vi "KN-StringTo矩形AndOptions.vi"(0 "String":string) -> (4 "ROI Descriptor":T5 {"Contours"."Type" items=["No Selection", "Point", "Line", "Rectangle", "Oval", "Polygon", "Freehand Region", "Annulus", "Unused2", "Unused3", "Broken Line", "Freehand Line", "Rotated Rectangle"]}, 6 "Option All":T4 {"Edge Options"."Edge Polarity" items=["All Edges", "Rising Edges", "Falling Edges"]; "Edge Options"."Minimum Edge Strength" format="%.2f"; "Edge Options"."Width" step=2; "Edge Options"."Kernel Size" step=2}, 8 "UI SHOW":T3 {"Edge Options"."Edge Polarity" items=["All Edges", "Rising Edges", "Falling Edges"]; "Edge Options"."Minimum Edge Strength" format="%.2f"; "Edge Options"."Width" step=2; "Edge Options"."Kernel Size" step=2}, 15 "Range (Threshold 1)":cluster{"Lower value":sgl, "Upper value":sgl}={"Lower value"=218.0, "Upper value"=255.0})   [LabVIEW 2015]
uses:
  <vilib>/vision/Measure.llb/Edge Options.ctl
  <vilib>/vision/Measure.llb/Edge Polarity.ctl
panel:
  out "已删除元素的数组子集":string[](array[string])
  out "已删除的部分":string[](array[string])
  out "All Data":string[](array[string])
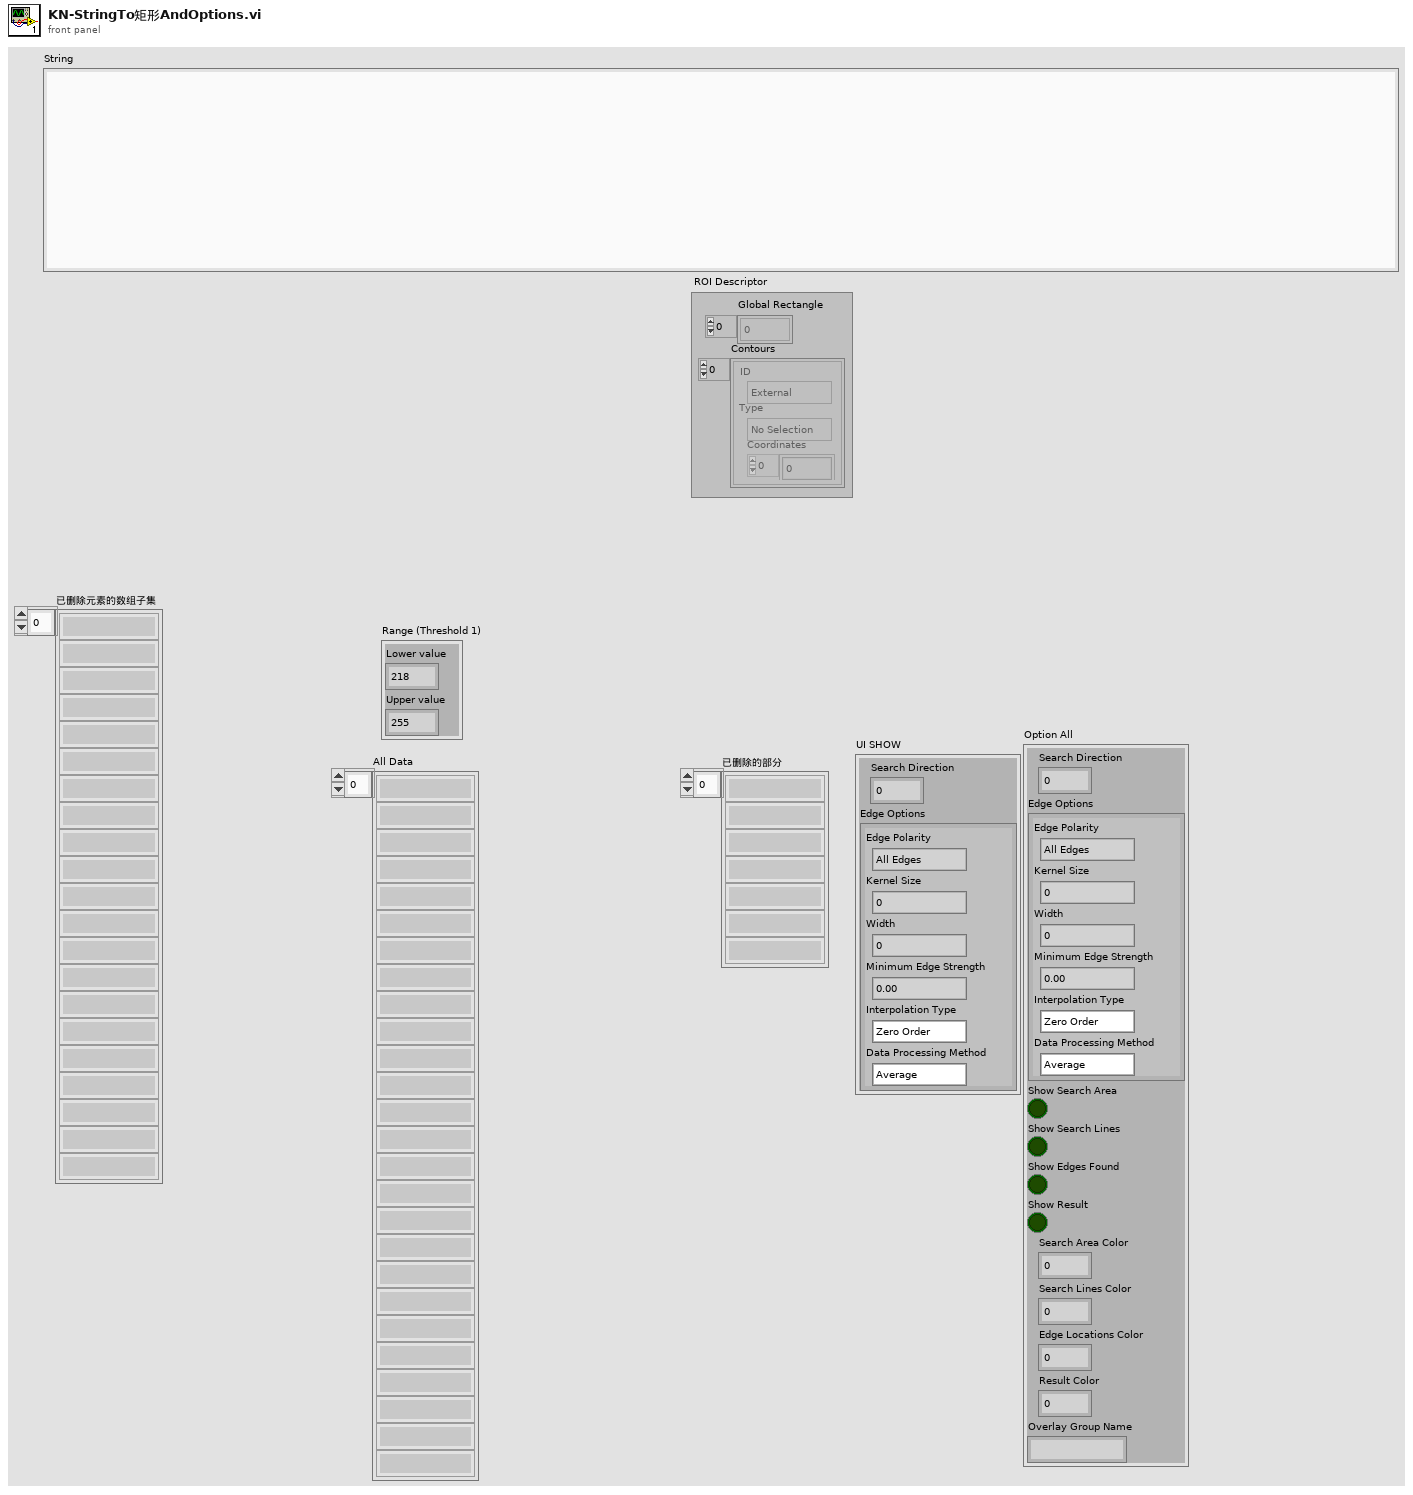
[diagram p1: front panel]
types:
  T1 = typedef "Edge Options.ctl" = cluster{"Edge Polarity":T2, "Kernel Size":u32, "Width":u32, "Minimum Edge Strength":sgl, "Interpolation Type":enum32{"Zero Order", "Bilinear", "Quadratic", "Cubic", "Bilinear Fixed"}, "Data Processing Method":enum32{"Average", "Median"}}
  T2 = typedef "Edge Polarity.ctl" = u32
  T3 = cluster{"Search Direction":u32, "Edge Options":T1}
  T4 = cluster{"Search Direction":u32, "Edge Options":T1, "Show Search Area":bool, "Show Search Lines":bool, "Show Edges Found":bool, "Show Result":bool, "Search Area Color":u32, "Search Lines Color":u32, "Edge Locations Color":u32, "Result Color":u32, "Overlay Group Name":string}
  T5 = typedef "ROI Descriptor" = cluster{"Global Rectangle":i32[], "Contours":cluster{"ID":enum32{"External", "Internal"}, "Type":u32, "Coordinates":i32[]}[]}
  T6 = typedef "IMAQ Rectangle" = cluster{"Left":i32, "Top":i32, "Right":i32, "Bottom":i32, "Rotation":dbl}
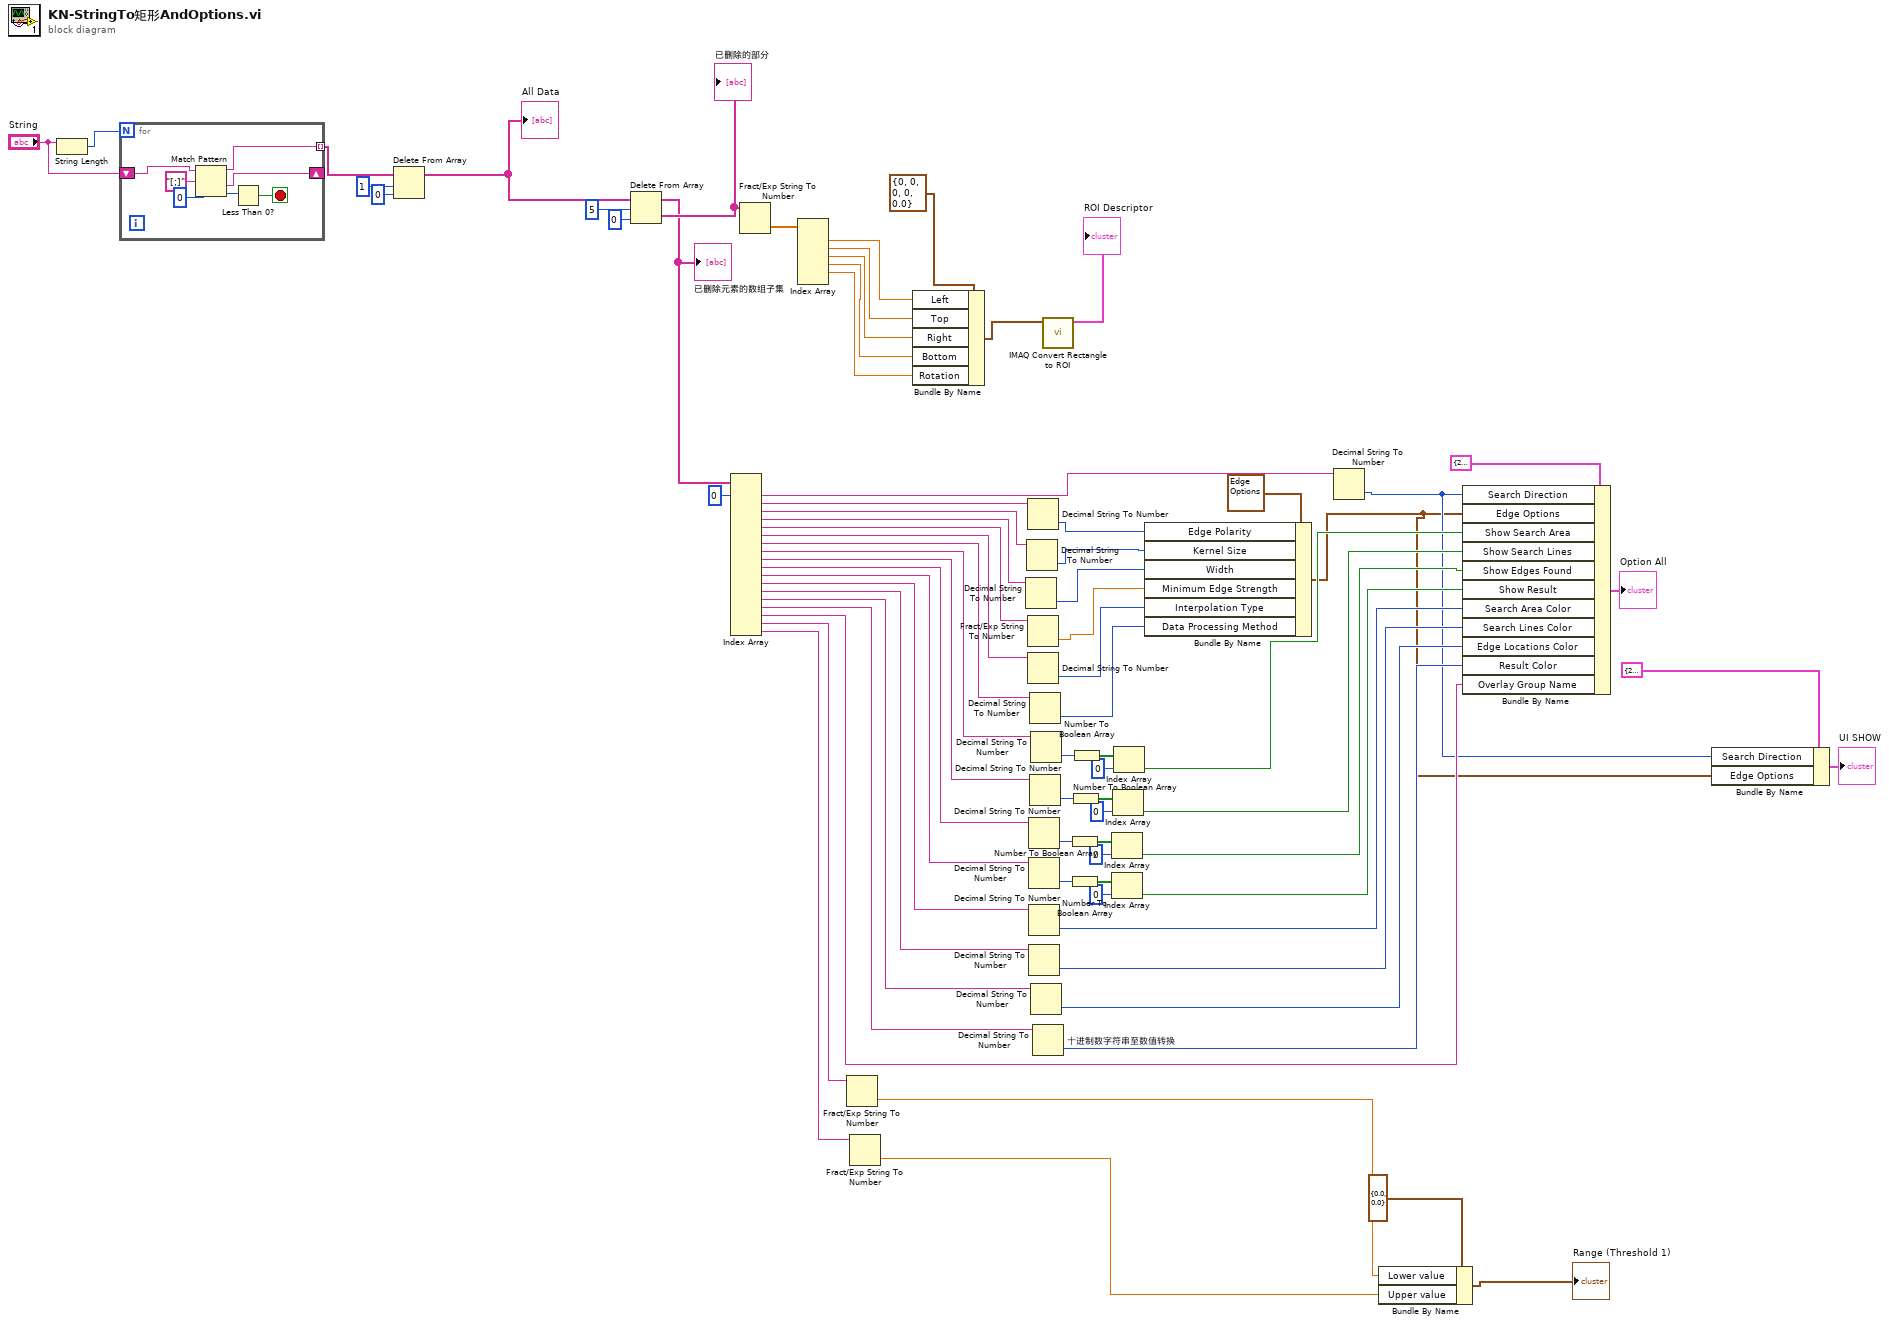
[diagram p0: block diagram]
diagram:
  n1 = String Length(string="String") -> (length=w74:i32)
  n2 = for {
    N: w74 -> [_]
    shift-right: [w77] -> _
    shift-left: "String" -> [w78]
    tunnel: [w76] -> w73 mode=indexing
    stop <- w79 stop-if-true
    n3 = Match Pattern(string=w78, regular expression="[;]" ("正则表达式"), offset (0)=0 ("偏移量(0)")) -> (before substring=w76:string, after substring=w77:string, offset past match=w80:i32)  [unwired: 1 out]
    n4 = Less Than 0?(x=w80) -> (x < 0?=w79:bool)
  }
  n5 = Delete From Array(array=w73, length=1 ("长度"), index=0 ("索引")) -> (array with subset deleted=w70:string[])  [unwired: 1 out]
  "All Data" <- w70
  n6 = Delete From Array(array=w70, length=5 ("长度"), index=0 ("索引")) -> (deleted portion=w67:string[], array with subset deleted=w64:string[])
  "已删除的部分" <- w67
  "已删除元素的数组子集" <- w64
  n7 = Index Array(array=w64, index #1=0 ("索引")) -> (element #1=w60:string, element #2=w59:string, element #3=w57:string, element #4=w55:string, element #5=w53:string, element #6=w51:string, element #7=w50:string, element #8=w47:string, element #9=w34:string, element #10=w33:string, element #11=w32:string, element #12=w28:string, element #13=w27:string, element #14=w26:string, element #15=w25:string, element #16=w20:string, element #17=w4:string, element #18=w3:string)  [unwired: 17 in]
  n8 = Fract/Exp String To Number(string=w67) -> (number=w66:dbl[])  [unwired: 3 in, 1 out]
  n9 = Index Array(array=w66) -> (element #1=w18:dbl, element #2=w17:dbl, element #3=w19:dbl, element #4=w16:dbl, element #5=w65:dbl)  [unwired: 6 in, 1 out]
  n10 = Fract/Exp String To Number(string=w4) -> (number=w13:dbl)  [unwired: 3 in, 1 out]
  n11 = Fract/Exp String To Number(string=w3) -> (number=w12:dbl)  [unwired: 3 in, 1 out]
  n12 = Bundle By Name(cluster=T6 {"Left"=0, "Top"=0, "Right"=0, "Bottom"=0, "Rotation"=0.0} ("Rectangle"), "Left"=w18, "Top"=w17, "Right"=w19, "Bottom"=w16, "Rotation"=w65) -> (w6:T6)
  n13 = Decimal String To Number(string=w55) -> (number=w54:i32)  [unwired: 2 in, 1 out]
  n14 = Decimal String To Number(string=w57) -> (number=w56:i32)  [unwired: 2 in, 1 out]
  n15 = Decimal String To Number(string=w59) -> (number=w58:i32)  [unwired: 2 in, 1 out]
  n16 = Fract/Exp String To Number(string=w53) -> (number=w52:dbl)  [unwired: 3 in, 1 out]
  n17 = Decimal String To Number(string=w51) -> (number=w49:i32)  [unwired: 2 in, 1 out]
  n18 = Decimal String To Number(string=w33) -> (number=w40:i32)  [unwired: 2 in, 1 out]
  n19 = Decimal String To Number(string=w32) -> (number=w35:i32)  [unwired: 2 in, 1 out]
  n20 = Decimal String To Number(string=w28) -> (number=w24:i32)  [unwired: 2 in, 1 out]
  n21 = Decimal String To Number(string=w27) -> (number=w23:i32)  [unwired: 2 in, 1 out]
  n22 = Decimal String To Number(string=w50) -> (number=w48:i32)  [unwired: 2 in, 1 out]
  n23 = Decimal String To Number(string=w34) -> (number=w41:i32)  [unwired: 2 in, 1 out]
  n24 = Decimal String To Number(string=w47) -> (number=w46:i32)  [unwired: 2 in, 1 out]
  n25 = Decimal String To Number(string=w26) -> (number=w22:i32)  [unwired: 2 in, 1 out]
  n26 = Decimal String To Number "十进制数字符串至数值转换"(string=w25) -> (number=w21:i32)  [unwired: 2 in, 1 out]
  n27 = call "IMAQ Convert Rectangle to ROI"("Rectangle"=w6) -> ("ROI Descriptor"=→"ROI Descriptor":T5)  [unwired: 8 in, 1 out]
  n28 = Number To Boolean Array(number=w40) -> (Boolean array=w39:bool[])
  n29 = Number To Boolean Array(number=w35) -> (Boolean array=w36:bool[])
  n30 = Number To Boolean Array(number=w41) -> (Boolean array=w42:bool[])
  n31 = Number To Boolean Array(number=w46) -> (Boolean array=w45:bool[])
  n32 = Index Array(array=w39, index=0 ("索引")) -> (element=w30:bool)
  n33 = Index Array(array=w36, index=0 ("索引")) -> (element=w29:bool)
  n34 = Index Array(array=w42, index=0 ("索引")) -> (element=w31:bool)
  n35 = Index Array(array=w45, index=0 ("索引")) -> (element=w15:bool)
  n36 = Bundle By Name(cluster=T1 {"Edge Polarity"=0, "Kernel Size"=0, "Width"=0, "Minimum Edge Strength"=0.0, "Interpolation Type"=enum."Bilinear Fixed", "Data Processing Method"=enum."Average"} ("Edge Options"), "Edge Polarity"=w58, "Kernel Size"=w56, "Width"=w54, "Minimum Edge Strength"=w52, "Interpolation Type"=w49, "Data Processing Method"=w48) -> (w8:T1)
  n37 = Decimal String To Number(string=w60) -> (number=w9:i32)  [unwired: 2 in, 1 out]
  n38 = Bundle By Name(cluster=cluster{"Lower value":sgl, "Upper value":sgl} {"Lower value"=0.0, "Upper value"=0.0} ("Red or Hue Range (Color Threshold 1)"), "Lower value"=w13, "Upper value"=w12) -> (→"Range (Threshold 1)":cluster{"Lower value":sgl, "Upper value":sgl})
  n39 = Bundle By Name(cluster=T4 {"Search Direction"=2, "Edge Options"={"Edge Polarity"=0, "Kernel Size"=0, "Width"=0, "Minimum Edge Strength"=0.0, "Interpolation Type"=enum."Bilinear Fixed", "Data Processing Method"=enum."Average"}, "Show Search Area"=FALSE, "Show Search Lines"=FALSE, "Show Edges Found"=FALSE, "Show Result"=TRUE, "Search Area Color"=65280, "Search Lines Color"=255, "Edge Locations Color"=16776960, "Result Color"=16711680, "Overlay Group Name"=""} ("Options (Find Circular Edge 1)"), "Search Direction"=w9, "Edge Options"=w8, "Show Search Area"=w15, "Show Search Lines"=w31, "Show Edges Found"=w30, "Show Result"=w29, "Search Area Color"=w24, "Search Lines Color"=w23, "Edge Locations Color"=w22, "Result Color"=w21, "Overlay Group Name"=w20) -> (→"Option All":T4)
  n40 = Bundle By Name(cluster=T3 {"Search Direction"=2, "Edge Options"={"Edge Polarity"=0, "Kernel Size"=0, "Width"=0, "Minimum Edge Strength"=0.0, "Interpolation Type"=enum."Bilinear Fixed", "Data Processing Method"=enum."Average"}} ("Options (Find Circular Edge 1)"), "Search Direction"=w9, "Edge Options"=w8) -> (→"UI SHOW":T3)
